vi "Edit.vi"(10 "Configuration":refnum<data-value>, 11 "LogicName":string) -> ()   [LabVIEW 2025, in "PLC_Module.lvlib" / "PLC_Module.lvclass"]
uses:
  PLC_Module.lvclass
  PLC_Data.ctl
  PLC_Data_Type.ctl
  PLC_Module.lvclass/PLC_Module.ctl
  <vilib>/addons/_JKI Toolkits/State Machine/_JKI_lib_State_Machine.llb/Select State(s)_err__jki_lib_state_machine.vi
  PLC_Data_Config.ctl
panel:
  in  "Cancel":bool
  in  "OK":bool
  in  "Config":T1
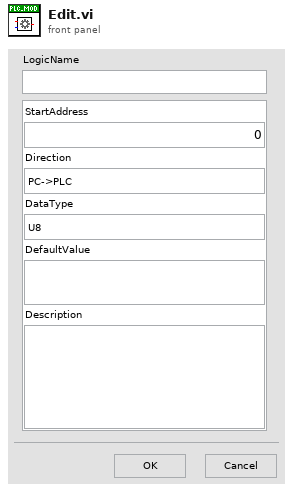
[diagram p1: front panel]
types:
  T1 = typedef "PLC_Module.lvlib/PLC_Module.lvclass/PLC_Data.ctl" = cluster{"StartAddress":u32, "Direction":enum16{"PC->PLC", "PLC->PC"}, "DataType":T2, "DefaultValue":string, "Description":string}
  T2 = typedef "PLC_Module.lvlib/PLC_Module.lvclass/PLC_Data_Type.ctl" = enum16{"U8", "U32", "U32_Array", "String"}
  T3 = enum32{"Invalid", "Standard", "Closed", "Hidden", "Minimized", "Maximized"}
  T4 = enum32{"invalid app kind", "Development System", "Run Time System", "Student Edition", "Embedded LabVIEW", "Evaluation", "Custom"}
  T5 = enum8{"Enabled", "Disabled", "Disabled and Grayed Out"}
  T6 = cluster{"Core":cluster{"Current VI Reference":refnum<vi>, "Close Panel on Exit?":bool}, "Configuration":refnum<data-value>, "LogicName":refnum<vi>, "Config":refnum<vi>}
  T7 = cluster{"Current VI Reference":refnum<vi>, "Close Panel on Exit?":bool}
  T8 = typedef "PLC_Module.lvlib/PLC_Module.lvclass/PLC_Data_Config.ctl" = map{string, cluster{"Config":T1, "Value":string}}
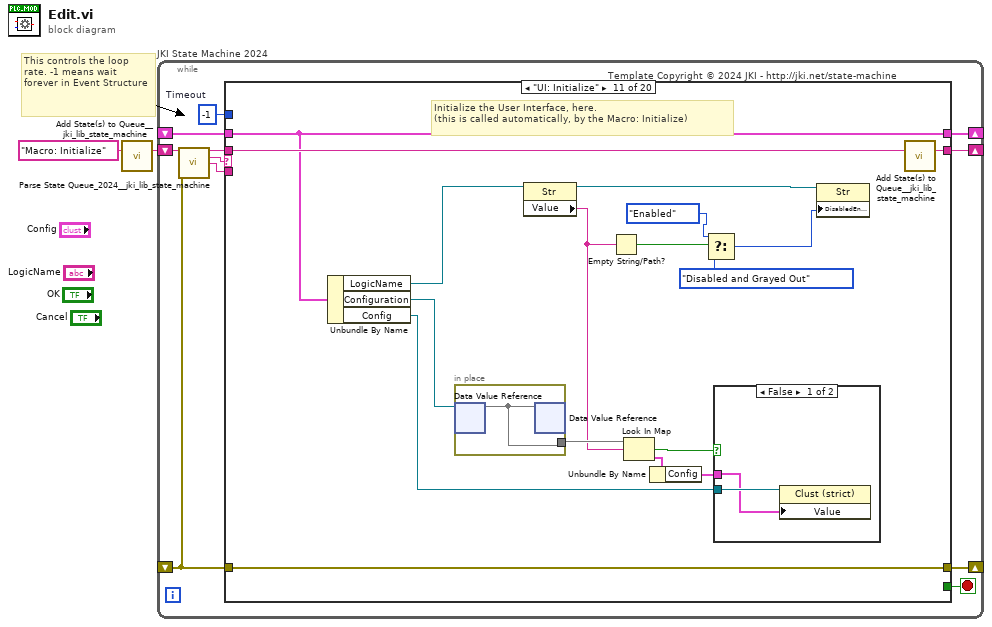
[diagram p0: block diagram]
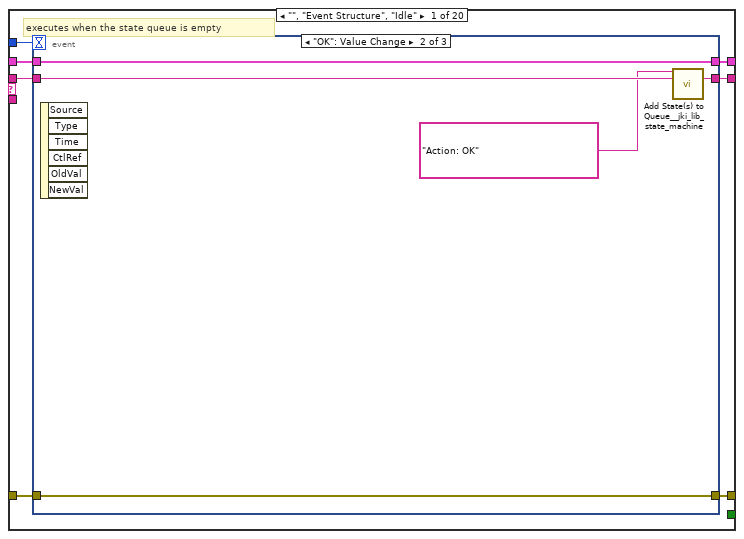
[diagram p2: hidden frame]
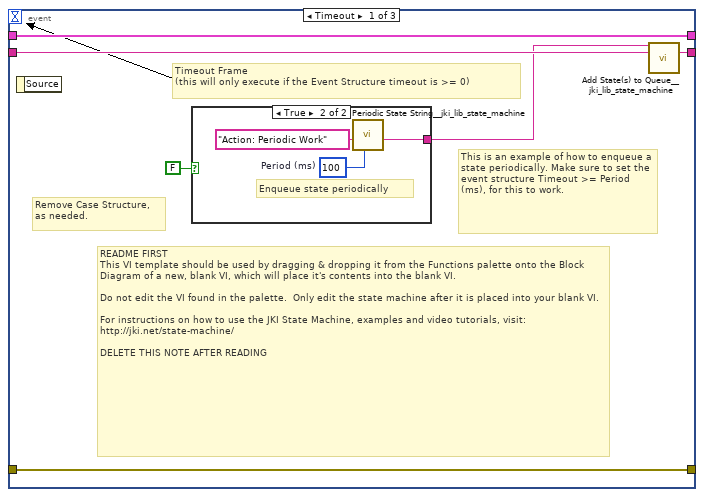
[diagram p3: hidden frame]
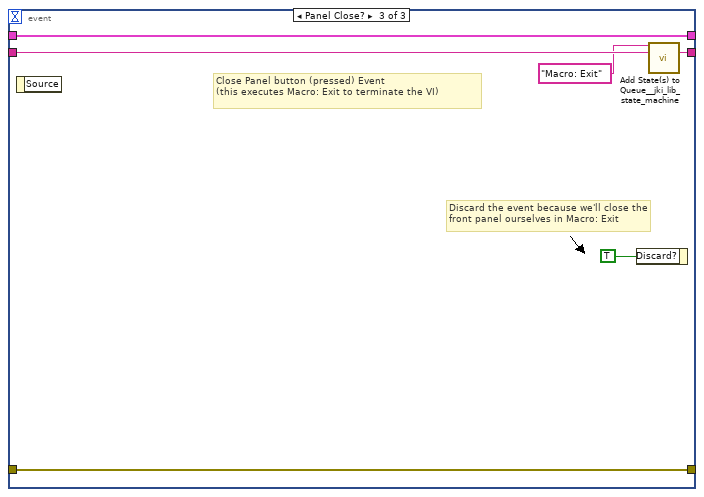
[diagram p5: hidden frame]
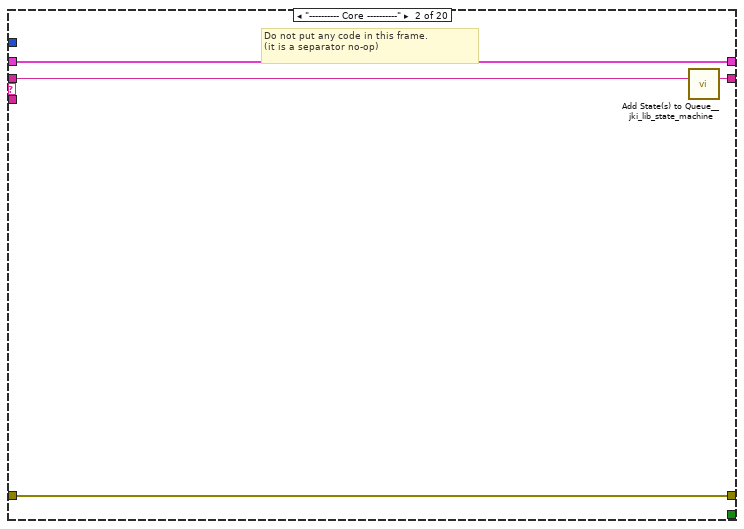
[diagram p6: hidden frame]
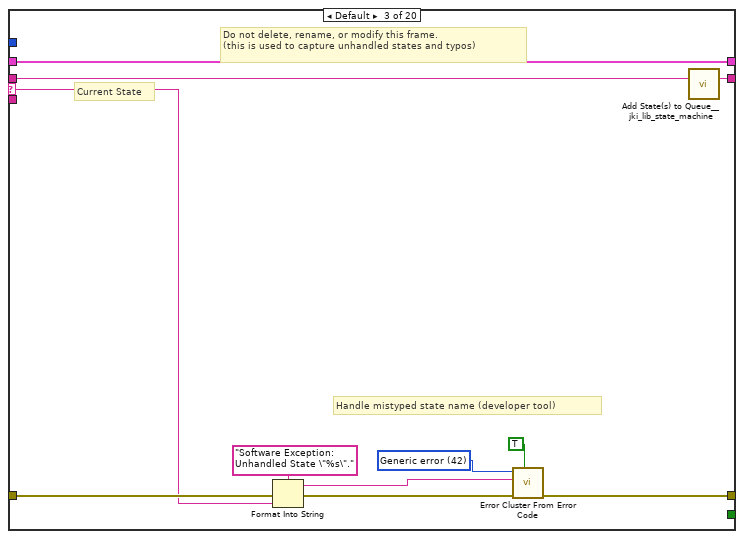
[diagram p7: hidden frame]
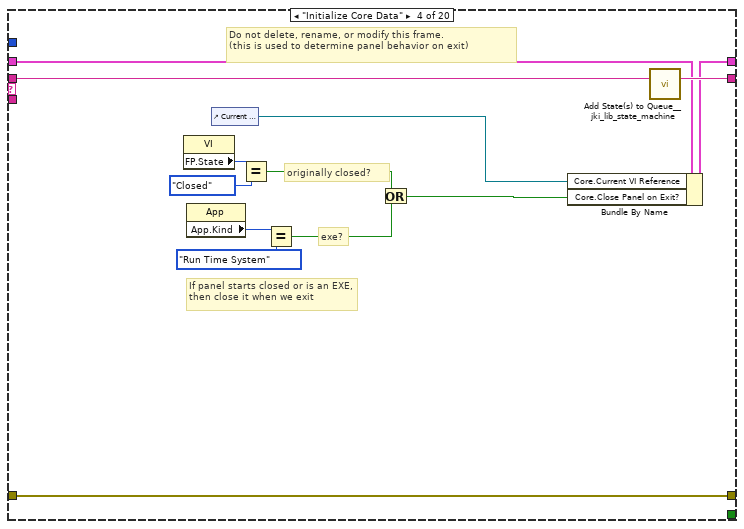
[diagram p8: hidden frame]
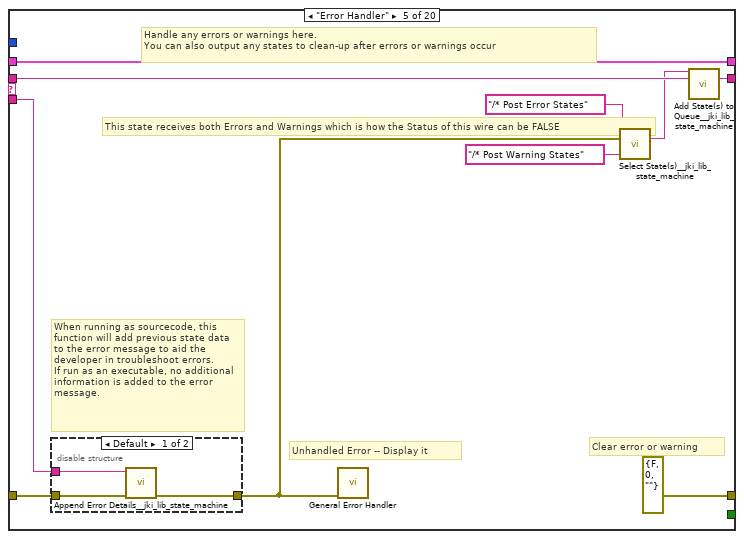
[diagram p9: hidden frame]
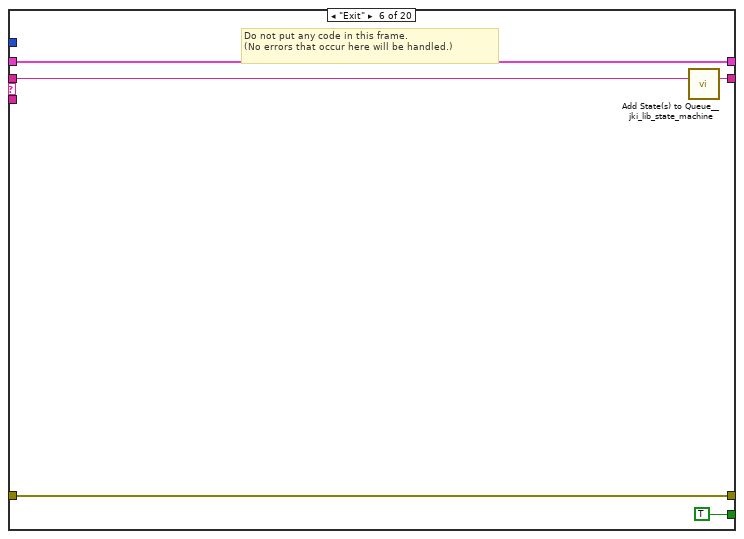
[diagram p11: hidden frame]
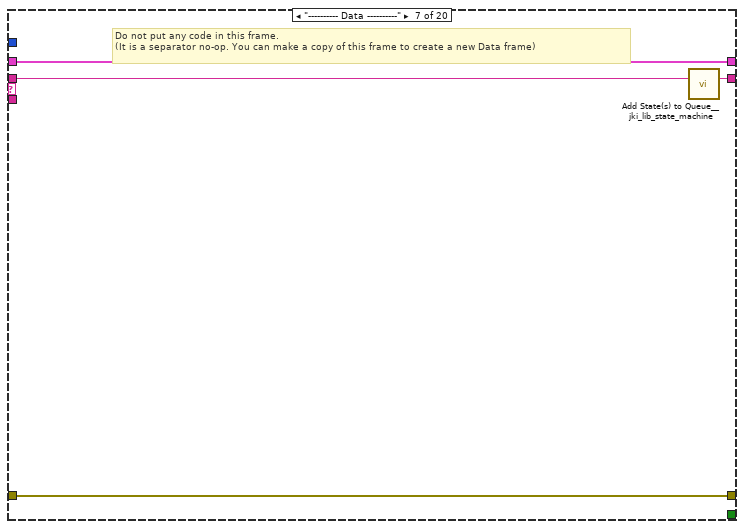
[diagram p12: hidden frame]
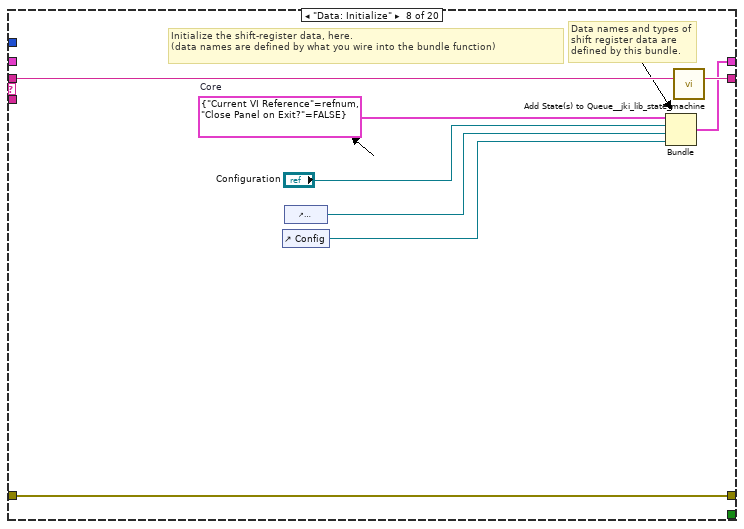
[diagram p13: hidden frame]
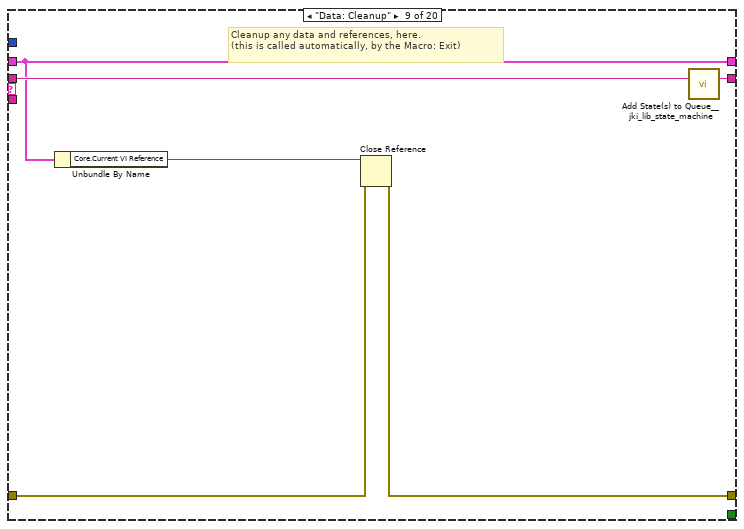
[diagram p14: hidden frame]
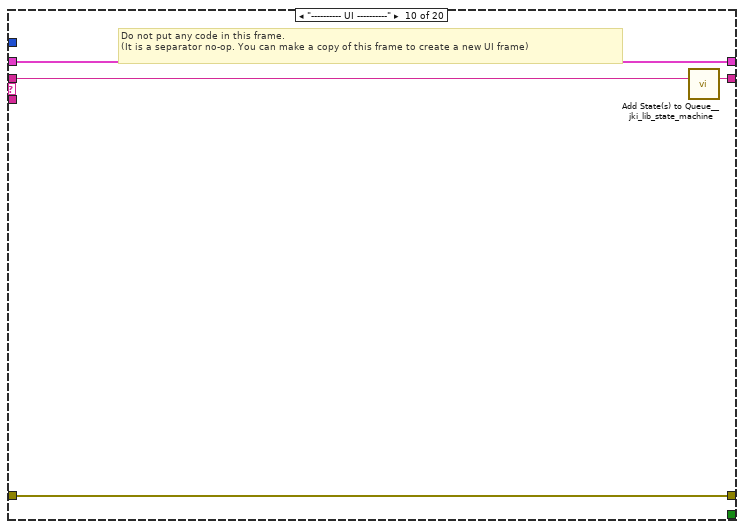
[diagram p15: hidden frame]
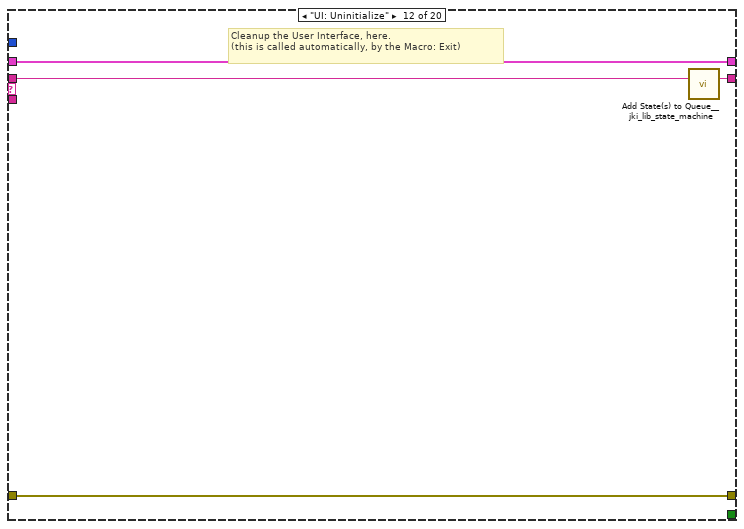
[diagram p17: hidden frame]
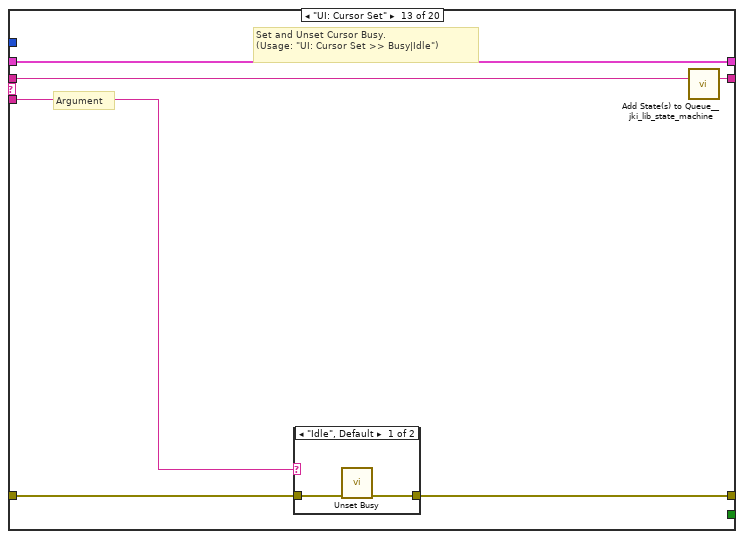
[diagram p18: hidden frame]
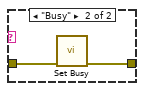
[diagram p19: hidden frame]
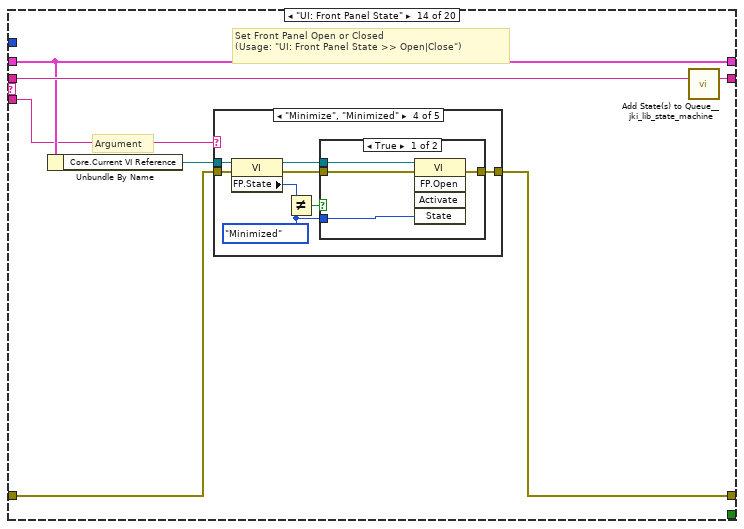
[diagram p20: hidden frame]
diagram:
  # "This controls the loop rate. -1 means wait forever in Event Structure"
  n1 = call <vilib>:"Add State(s) to Queue__jki_lib_state_machine.vi"("State(s) in (\"\")"="Macro: Initialize") -> ("States Out"=w2:string)  [unwired: 14 in]
  n2 = while "JKI State Machine 2024" {
    shift-right: [w6] -> _
    shift-left: _ -> [w5]
    shift-right: [w9] -> _
    shift-left: _ -> [w3]
    shift-right: [w8] -> _
    shift-left: w2 -> [w10]
    stop <- w7 stop-if-true
    w4 = -1  # Timeout
    # "Template Copyright © 2024 JKI - http://jki.net/state-machine"
    n3 = call <vilib>:"Parse State Queue_2024__jki_lib_state_machine.vi"("State Queue"=w10, "Error In (no error)"=w3) -> ("Remaining States"=w12:string, "Current State"=w13:string, "Arguments"=w11:string)  [unwired: 11 in]
    n4 = case shown="\"UI: Initialize\"" w13 {
      selector: w13 -> [_ _ w45 _ _ _ _ _ _ _ _ _ _ _ _ _ _ _ _ _]
      tunnel: w12 -> [w20 w44 w49 w68 w78 w87 w91 w99 w105 w109 w126 w133 w139 w150 w219 w224 w233 w237 w241 w245]
      tunnel: w11 -> [_ _ _ _ w73 _ _ _ _ _ _ _ w134 w144 _ _ _ _ _ _]
      tunnel: w5 -> [w18 w41 w47 w61 w75 w85 w88 _ w100 w106 w123 w131 w137 w146 w216 w221 w231 w234 w238 w242]
      tunnel: [w17 w42 w51 w65 errorcluster {"status"=FALSE, "code"=0, "source"=""} ("error out") w84 w89 w96 w101 w107 w124 w130 w135 w147 w217 w222 w228 w235 w239 w243] -> w9
      tunnel: w3 -> [w14 w42 w50 w65 w74 w84 w89 w96 w102 w107 w124 w130 w136 w148 w217 w222 w228 w235 w239 w243]
      tunnel: [w19 w43 w48 w67 w77 w86 w90 w98 w104 w108 w125 w132 w138 w149 w218 w223 w232 w236 w240 w244] -> w8
      tunnel: [_ _ _ _ _ TRUE _ _ _ _ _ _ _ _ _ _ _ _ _ _] -> w7
      tunnel: [w16 w41 w47 w66 w75 w85 w88 w97 w100 w106 w123 w131 w137 w146 w216 w221 w231 w234 w238 w242] -> w6
      tunnel: w4 -> [w15 _ _ _ _ _ _ _ _ _ _ _ _ _ _ _ _ _ _ _]
      frame "", "Event Structure", "Idle" {
        # "executes when the state queue is empty"
        n5 = event shown="[1] \"OK\": Value Change" {
          selector: _ -> [_ _ _]
          dyn-events: _ -> [_ _ _]
          timeout: w15 -> [_ _ _]
          tunnel: w20 -> [w26 w34 w40]
          tunnel: [w25 w33 w39] -> w19
          tunnel: w18 -> [w23 w31 w37]
          tunnel: [w24 w32 w38] -> w17
          tunnel: w14 -> [w24 w32 w38]
          tunnel: [w23 w31 w37] -> w16
          event Timeout {
            # "Remove Case Structure, as needed."
            # "This is an example of how to enqueue a state periodically. Make sure to set the event structure Timeout >= Period (ms), for this to work."
            # "README FIRST\nThis VI template should be used by dragging & dropping it from the Functions palette onto the Block Diagram of a new, blank VI, which will place it's contents into the blank VI.\n\nDo not edit the VI found in the palette.  Only edit the state machine after it is placed into your blank VI.\n\nFor instructions on how to use the JKI State Machine, examples and video tutorials, visit:\nhttp://jki.net/state-machine/\n\nDELETE THIS NOTE AFTER READING"
            # "Timeout Frame\n(this will only execute if the Event Structure timeout is >= 0)"
            n6 = event-data() -> ()  [unwired: 1 in, 1 out]
            n7 = case shown="True" FALSE {
              tunnel: [_ w29] -> w22
              frame False {
              }
              frame True {
                w27 = u32 100  # Period (ms)
                # "Enqueue state periodically"
                n8 = call <vilib>:"Periodic State String__jki_lib_state_machine.vi"("Period (ms)"=w27, "State"="Action: Periodic Work") -> ("State Out"=w29:string)  [unwired: 9 in]
              }
            }
            n9 = call <vilib>:"Add State(s) to Queue__jki_lib_state_machine.vi"("State(s) in Front (\"\")"=w22, "State(s) in (\"\")"=w26) -> ("States Out"=w25:string)  [unwired: 13 in]
          }
          event "OK": Value Change {
            n10 = event-data() -> ()  [unwired: 1 in, 6 out]
            n11 = call <vilib>:"Add State(s) to Queue__jki_lib_state_machine.vi"("State(s) in Front (\"\")"="Action: OK" ("State(s) in Front (\"\")"), "State(s) in (\"\")"=w34) -> ("States Out"=w33:string)  [unwired: 13 in]
          }
          event Panel Close? {
            # "Discard the event because we'll close the front panel ourselves in Macro: Exit"
            # "Close Panel button (pressed) Event\n(this executes Macro: Exit to terminate the VI)"
            n12 = event-data() -> ()  [unwired: 1 in, 1 out]
            n13 = event-data("Discard?"=TRUE) -> ()  [unwired: 1 in, 1 out]
            n14 = call <vilib>:"Add State(s) to Queue__jki_lib_state_machine.vi"("State(s) in Front (\"\")"="Macro: Exit", "State(s) in (\"\")"=w40) -> ("States Out"=w39:string)  [unwired: 13 in]
          }
        }
      }
      frame "---------- Core ----------" {
        # "Do not put any code in this frame.\n(it is a separator no-op)"
        n15 = call <vilib>:"Add State(s) to Queue__jki_lib_state_machine.vi"("State(s) in (\"\")"=w44) -> ("States Out"=w43:string)  [unwired: 14 in]
      }
      frame Default {
        w54 = 42 items=["No error", "Argument error", "Memory is full", "Out of zone", "End of file", "File already open", "Generic file I/O error", "File not found", "File permission error", "Disk is full", "Duplicate path", "Too many files open", "System feature not enabled", "Resource file not found", "Cannot add resource", "Resource not found", "Image not found", "Image memory error", "Pen does not exist", "Config type invalid", "Config token not found", "Config parse error", "Config memory error", "Bad external code format", "Bad external code offset", "External code not present", "Null window", "Destroy window error", "Null menu", "Print aborted", "Bad print record", "Print driver error", "Windows error during printing", "Memory error during printing", "Print dialog error", "Generic print error", "Invalid device refnum", "Device not found", "Device parameter error", "Device unit error", "Cannot open device", "Device call aborted", "Generic error", "Cancelled by user", "Object ID too low", "Object ID too high", "Object not in heap", "Unknown heap", "Unknown object (invalid DefProc)", "Unknown object (DefProc not in table)", "Message out of range", "Invalid (null) method", "Unknown message", "Manager call not supported", "Bad address", "Network operation in progress", "Network operation timed out", "Connection is busy", "Network attribute not supported", "Network error", "Address in use", "System out of memory", "Connection aborted", "Connection refused", "Not connected", "Already connected", "Connection closed", "Initialization error (interapplication manager)", "Bad occurrence", "Wait on unbound occurrence handler", "Occurrence queue overflow", "Datalog type conflict", "Unused", "Unrecognized type (interapplication manager)", "Memory corrupt", "Failed to make temporary DLL", "Old CIN version", "Drag socket not found", "Failed to load drop-object", "Failed to register OLE object", "Failed to release OLE object", "Format specifier type mismatch", "Unknown format specifier", "Too few format specifiers", "Too many format specifiers", "Scan failed", "Newer CIN version", "Error converting to variant", "Runtime menu error", "Password tampered", "Variant attribute not found", "Incompatible variant data type", "Event data is not available", "Event Store is not present", "Occurrence is not found", "Event Queue is not created", "Event info is not available", "Refnum passed is NULL", "Error retrieving Class GUID", "Error retrieving CoClass GUID", "Error retrieving TypeLib GUID.", "Bad built application magic bytes.", "Specific driver is different from the specific driver associated with the Logical Name.", "There is no session opened to the class driver.", "Max Error", "MAX - Error with config objects", "MAX - Error loading configuration", "MAX - Group not supported"]
        # "Current State"
        # "Do not delete, rename, or modify this frame.\n(this is used to capture unhandled states and typos)"
        # "Handle mistyped state name (developer tool)"
        n16 = Format Into String(format string="Software Exception: Unhandled State \"%s\"." ("message"), error in=w50, w45) -> (resulting string=w53:string, error out=w52:errorcluster)  [unwired: 1 in]
        n17 = call <vilib>:"Error Cluster From Error Code.vi"("show call chain? (False)"=TRUE, "error in (no error)"=w52, "error message (\"\")"=w53, "error code (0)"=w54) -> ("error out"=w51:errorcluster)  [unwired: 5 in]
        n18 = call <vilib>:"Add State(s) to Queue__jki_lib_state_machine.vi"("State(s) in (\"\")"=w49) -> ("States Out"=w48:string)  [unwired: 14 in]
      }
      frame "Initialize Core Data" {
        # "Do not delete, rename, or modify this frame.\n(this is used to determine panel behavior on exit)"
        # "originally closed?"
        # "exe?"
        # "If panel starts closed or is an EXE, then close it when we exit"
        n19 = property class="VI"() -> ("FP.State"=w58:T3)  [unwired: 2 in, 2 out]
        n20 = property class="App"() -> ("App.Kind"=w64:T4)  [unwired: 2 in, 2 out]
        n21 = control-ref of="Current VI Reference"() -> (w59:refnum<vi>)
        n22 = Equal?(x=w58, y=T3."Closed" ("Front Panel Window:State")) -> (x = y?=w56:bool)
        n23 = Equal?(x=w64, y=T4."Run Time System" ("Application:Kind")) -> (x = y?=w62:bool)
        n24 = Or(x=w56, y=w62) -> (x .or. y?=w60:bool)
        n25 = Bundle By Name(cluster=w61, "Core.Current VI Reference"=w59, "Core.Close Panel on Exit?"=w60) -> (w66:T6)
        n26 = call <vilib>:"Add State(s) to Queue__jki_lib_state_machine.vi"("State(s) in (\"\")"=w68) -> ("States Out"=w67:string)  [unwired: 14 in]
      }
      frame "Error Handler" {
        # "When running as sourcecode, this function will add previous state data to the error message to aid the developer in troubleshoot errors.\nIf run as an executable, no additional information is added to the error message."
        # "This state receives both Errors and Warnings which is how the Status of this wire can be FALSE"
        # "Unhandled Error -- Display it"
        # "Handle any errors or warnings here.\nYou can also output any states to clean-up after errors or warnings occur"
        # "Clear error or warning"
        n27 = disable-structure shown="Default" {
          disable-tunnel: w74 -> [w81 w82]
          disable-tunnel: w73 -> [w80 _]
          disable-tunnel: [w79 w82] -> w72
          frame condition #0 (active) {
            n28 = call <vilib>:"Append Error Details__jki_lib_state_machine.vi"("error in (no error)"=w81, "Previous State and Argument(s)"=w80) -> ("error out"=w79:errorcluster)  [unwired: 9 in]
          }
          frame condition #1 {
          }
        }
        n29 = call <vilib>:"General Error Handler.vi"("error in (no error)"=w72) -> ()  [unwired: 10 in, 5 out]
        n30 = call-poly <vilib>:"Select State(s)__jki_lib_state_machine.vi"("State(s) if True (\"\")"="/* Post Error States", "Select"=w72, "State(s) if False (\"\")"="/* Post Warning States") -> ("States Out"=w70:string)  [unwired: 12 in]
        n31 = call <vilib>:"Add State(s) to Queue__jki_lib_state_machine.vi"("State(s) in Front (\"\")"=w70, "State(s) in (\"\")"=w78) -> ("States Out"=w77:string)  [unwired: 13 in]
      }
      frame "Exit" {
        # "Do not put any code in this frame.\n(No errors that occur here will be handled.)"
        n32 = call <vilib>:"Add State(s) to Queue__jki_lib_state_machine.vi"("State(s) in (\"\")"=w87) -> ("States Out"=w86:string)  [unwired: 14 in]
      }
      frame "---------- Data ----------" {
        # "Do not put any code in this frame.\n(It is a separator no-op. You can make a copy of this frame to create a new Data frame)"
        n33 = call <vilib>:"Add State(s) to Queue__jki_lib_state_machine.vi"("State(s) in (\"\")"=w91) -> ("States Out"=w90:string)  [unwired: 14 in]
      }
      frame "Data: Initialize" {
        w95 = T7 {"Current VI Reference"=refnum, "Close Panel on Exit?"=FALSE}  # Core
        # "Data names and types of shift register data are defined by this bundle."
        # "Initialize the shift-register data, here.\n(data names are defined by what you wire into the bundle function)"
        n34 = control-ref of="Config"() -> (w92:refnum<vi>)
        n35 = control-ref of="LogicName"() -> (w93:refnum<vi>)
        n36 = Bundle("Core"=w95, "Configuration"="Configuration", "LogicName"=w93, "Config"=w92) -> (w97:T6)  [unwired: 1 in]
        n37 = call <vilib>:"Add State(s) to Queue__jki_lib_state_machine.vi"("State(s) in (\"\")"=w99) -> ("States Out"=w98:string)  [unwired: 14 in]
      }
      frame "Data: Cleanup" {
        # "Cleanup any data and references, here.\n(this is called automatically, by the Macro: Exit)"
        n38 = Unbundle By Name(w100) -> ("Core.Current VI Reference"=w103:refnum<vi>)
        n39 = Close Reference(reference=w103, error in (no error)=w102) -> (error out=w101:errorcluster)
        n40 = call <vilib>:"Add State(s) to Queue__jki_lib_state_machine.vi"("State(s) in (\"\")"=w105) -> ("States Out"=w104:string)  [unwired: 14 in]
      }
      frame "---------- UI ----------" {
        # "Do not put any code in this frame.\n(It is a separator no-op. You can make a copy of this frame to create a new UI frame)"
        n41 = call <vilib>:"Add State(s) to Queue__jki_lib_state_machine.vi"("State(s) in (\"\")"=w109) -> ("States Out"=w108:string)  [unwired: 14 in]
      }
      frame "UI: Initialize" {
        # "Initialize the User Interface, here.\n(this is called automatically, by the Macro: Initialize)"
        n42 = Unbundle By Name(w123) -> ("LogicName"=w122:refnum<vi>, "Configuration"=w116:refnum<data-value>, "Config"=w111:refnum<vi>)
        n43 = in-place {
          in-place-border: [w129] -> w115
          n44 = in-place-dvr #1(w116) -> (w129:T8)  [unwired: 1 out]
          n45 = in-place-dvr #1(w129) -> ()  [unwired: 2 out]
        }
        n46 = property class="Str"(reference=w122) -> (reference out=w121:refnum<vi>, "Value"=w114:string)  [unwired: 1 in, 1 out]
        n47 = Empty String/Path?(string/path=w114) -> (empty?=w120:bool)
        n48 = Look In Map(map=w115, key=w114) -> (key not found?=w113:bool, value=w112:cluster{"Config":T1, "Value":string})  [unwired: 1 in]
        n49 = Unbundle By Name(w112) -> ("Config"=w110:T1)
        n50 = Select(t=T5."Enabled" ("Disabled"), s=w120, f=T5."Disabled and Grayed Out") -> (s? t:f=w117:T5)
        n51 = case shown="False" w113 {
          tunnel: w110 -> [w127 _]
          tunnel: w111 -> [w128 _]
          frame False {
            n52 = property class="Clust (strict)"(reference=w128, "Value"=w127) -> ()  [unwired: 1 in, 2 out]
          }
          frame True {
          }
        }
        n53 = property class="Str"(reference=w121, "DisabledEnum"=w117) -> ()  [unwired: 1 in, 2 out]
        n54 = call <vilib>:"Add State(s) to Queue__jki_lib_state_machine.vi"("State(s) in (\"\")"=w126) -> ("States Out"=w125:string)  [unwired: 14 in]
      }
      frame "UI: Uninitialize" {
        # "Cleanup the User Interface, here.\n(this is called automatically, by the Macro: Exit)"
        n55 = call <vilib>:"Add State(s) to Queue__jki_lib_state_machine.vi"("State(s) in (\"\")"=w133) -> ("States Out"=w132:string)  [unwired: 14 in]
      }
      frame "UI: Cursor Set" {
        # "Argument"
        # "Set and Unset Cursor Busy.\n(Usage: \"UI: Cursor Set >> Busy|Idle\")"
        n56 = case shown="\"Idle\", Default" w134 {
          tunnel: w136 -> [w141 w143]
          tunnel: [w140 w142] -> w135
          frame "Idle", Default {
            n57 = call <vilib>:"Unset Busy.vi"("error in (no error)"=w141) -> ("error out"=w140:errorcluster)  [unwired: 10 in]
          }
          frame "Busy" {
            n58 = call <vilib>:"Set Busy.vi"("error in (no error)"=w143) -> ("error out"=w142:errorcluster)  [unwired: 9 in, 1 out]
          }
        }
        n59 = call <vilib>:"Add State(s) to Queue__jki_lib_state_machine.vi"("State(s) in (\"\")"=w139) -> ("States Out"=w138:string)  [unwired: 14 in]
      }
      frame "UI: Front Panel State" {
        # "Argument"
        # "Set Front Panel Open or Closed\n(Usage: \"UI: Front Panel State >> Open|Close\")"
        n60 = Unbundle By Name(w146) -> ("Core.Current VI Reference"=w145:refnum<vi>)
        n61 = case shown="\"Minimize\", \"Minimized\"" w144 {
          tunnel: w148 -> [w156 w171 w182 w195 w208]
          tunnel: [w158 w172 w184 w197 w210] -> w147
          tunnel: w145 -> [w157 w169 w183 w196 w209]
          frame "Open", "Standard", Default {
            w151 = T3."Standard" ("State")
            n62 = property class="VI"(reference=w157, error in=w156) -> (reference out=w154:refnum<vi>, error out=w155:errorcluster, "FP.State"=w153:T3)
            n63 = Not Equal?(x=w153, y=w151) -> (x != y?=w152:bool)
            n64 = case shown="True" w152 {
              tunnel: [w162 w164] -> w158
              tunnel: w155 -> [w161 w164]
              tunnel: w154 -> [w160 _]
              tunnel: w151 -> [w159 _]
              frame True {
                n65 = invoke class="VI" method="FP.Open"(reference=w160, error in=w161, "Activate"=TRUE, "State"=w159) -> (error out=w162:errorcluster)  [unwired: 1 in, 4 out]
              }
              frame False {
              }
            }
          }
          frame "Close", "Closed" {
            n66 = property class="VI"(reference=w169, error in=w171) -> (reference out=w168:refnum<vi>, error out=w170:errorcluster, "FP.State"=w166:T3)
            n67 = Not Equal?(x=w166, y=T3."Closed" ("Front Panel Window:State")) -> (x != y?=w165:bool)
            n68 = case shown="True" w165 {
              tunnel: [w173 w176] -> w172
              tunnel: w170 -> [w173 w175]
              tunnel: w168 -> [_ w174]
              frame False {
              }
              frame True {
                n69 = invoke class="VI" method="FP.Close"(reference=w174, error in=w175) -> (error out=w176:errorcluster)  [unwired: 1 in, 2 out]
              }
            }
          }
          frame "Hidden", "Hide" {
            w177 = T3."Hidden" ("State")
            n70 = property class="VI"(reference=w183, error in=w182) -> (reference out=w180:refnum<vi>, error out=w181:errorcluster, "FP.State"=w179:T3)
            n71 = Not Equal?(x=w179, y=w177) -> (x != y?=w178:bool)
            n72 = case shown="True" w178 {
              tunnel: [w188 w189] -> w184
              tunnel: w181 -> [w187 w189]
              tunnel: w180 -> [w186 _]
              tunnel: w177 -> [w185 _]
              frame True {
                n73 = invoke class="VI" method="FP.Open"(reference=w186, error in=w187, "State"=w185) -> (error out=w188:errorcluster)  [unwired: 2 in, 4 out]
              }
              frame False {
              }
            }
          }
          frame "Minimize", "Minimized" {
            w190 = T3."Minimized" ("State")
            n74 = property class="VI"(reference=w196, error in=w195) -> (reference out=w193:refnum<vi>, error out=w194:errorcluster, "FP.State"=w192:T3)
            n75 = Not Equal?(x=w192, y=w190) -> (x != y?=w191:bool)
            n76 = case shown="True" w191 {
              tunnel: [w201 w202] -> w197
              tunnel: w194 -> [w200 w202]
              tunnel: w193 -> [w199 _]
              tunnel: w190 -> [w198 _]
              frame True {
                n77 = invoke class="VI" method="FP.Open"(reference=w199, error in=w200, "State"=w198) -> (error out=w201:errorcluster)  [unwired: 2 in, 4 out]
              }
              frame False {
              }
            }
          }
          frame "Maximize", "Maximized" {
            w203 = T3."Maximized" ("State")
            n78 = property class="VI"(reference=w209, error in=w208) -> (reference out=w206:refnum<vi>, error out=w207:errorcluster, "FP.State"=w205:T3)
            n79 = Not Equal?(x=w205, y=w203) -> (x != y?=w204:bool)
            n80 = case shown="True" w204 {
              tunnel: [w214 w215] -> w210
              tunnel: w207 -> [w213 w215]
              tunnel: w206 -> [w212 _]
              tunnel: w203 -> [w211 _]
              frame True {
                n81 = invoke class="VI" method="FP.Open"(reference=w212, error in=w213, "State"=w211) -> (error out=w214:errorcluster)  [unwired: 2 in, 4 out]
              }
              frame False {
              }
            }
          }
        }
        n82 = call <vilib>:"Add State(s) to Queue__jki_lib_state_machine.vi"("State(s) in (\"\")"=w150) -> ("States Out"=w149:string)  [unwired: 14 in]
      }
      frame "---------- Macro ----------" {
        # "Do not put any code in this frame.\n(It is a separator no-op. You can make a copy of this frame to create a new Macro frame)"
        n83 = call <vilib>:"Add State(s) to Queue__jki_lib_state_machine.vi"("State(s) in (\"\")"=w219) -> ("States Out"=w218:string)  [unwired: 14 in]
      }
      frame "Macro: Initialize" {
        w220 = "Data: Initialize\nInitialize Core Data\nUI: Initialize\nUI: Front Panel State >> Open"  # Data: Initialize Initialize Core Data UI: Initialize UI: Front Panel State >> Open
        # "Initialization Macro\n(This is called once, when the VI starts)"
        n84 = call <vilib>:"Add State(s) to Queue__jki_lib_state_machine.vi"("State(s) in Front (\"\")"=w220, "State(s) in (\"\")"=w224) -> ("States Out"=w223:string)  [unwired: 13 in]
      }
      frame "Macro: Exit" {
        # "Exit Macro\n(This is called once, when the VI exits)"
        n85 = Unbundle By Name(w231) -> ("Core.Close Panel on Exit?"=w226:bool)
        n86 = call <vilib>:"Conditional State String__jki_lib_state_machine.vi"("Do State(s)?"=w226, "State"="UI: Front Panel State >> Close") -> ("State Out"=w225:string)  [unwired: 7 in]
        n87 = call <vilib>:"Add State(s) to Queue__jki_lib_state_machine.vi"("State(s) in (\"\")"=w225, "State(s) at Back (\"\")"="UI: Uninitialize\nData: Cleanup\nExit") -> ("States Out"=w229:string)  [unwired: 13 in]
        n88 = call <vilib>:"Add State(s) to Queue__jki_lib_state_machine.vi"("State(s) in Front (\"\")"=w229, "State(s) in (\"\")"=w233) -> ("States Out"=w232:string)  [unwired: 13 in]
      }
      frame "---------- Action ----------" {
        # "Template Separator\n(You can make a copy of, or modify, this frame)"
        n89 = call <vilib>:"Add State(s) to Queue__jki_lib_state_machine.vi"("State(s) in (\"\")"=w237) -> ("States Out"=w236:string)  [unwired: 14 in]
      }
      frame "Action: OK" {
        # "Your code here.\n(You can make a copy of, or modify, this frame)"
        n90 = call <vilib>:"Add State(s) to Queue__jki_lib_state_machine.vi"("State(s) in (\"\")"=w241) -> ("States Out"=w240:string)  [unwired: 14 in]
      }
      frame "Action: Cancel" {
        # "Your code here.\n(You can make a copy of, or modify, this frame)"
        n91 = call <vilib>:"Add State(s) to Queue__jki_lib_state_machine.vi"("State(s) in (\"\")"=w245) -> ("States Out"=w244:string)  [unwired: 14 in]
      }
    }
  }
